vi "Reset (uSMC).vi"(7 "Timeout (sec)":dbl=10.0, 8 "error in":errorcluster, 9 "Index":i32, 10 "Reset Direction (false - towards maximal value)":bool, 11 "Visa Array In":refnum<visa-resource-name>[](array[refnum])) -> (0 "error out":errorcluster, 3 "Visa Array Out":refnum<visa-resource-name>[](array[refnum]))   [LabVIEW 2010, in "SignalWriterMH110203USBStepperMotor.lvclass"]
uses:
  SignalWriterMH110203USBStepperMotor.lvclass
  class_data.vi
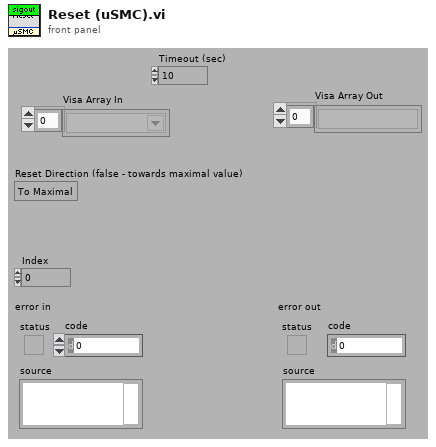
[diagram p1: front panel]
types:
  T1 = typedef "SignalWriterMH110203USBStepperMotor.lvclass/GoTo Control (uSMC).ctl" = cluster{"Step motor ID":string, "SMname":string, "Backlash":u16, "wait for input sygnal to start":bool, "use slow start/stop":bool, "units name":string, "Maximum speed":dbl, "speed":dbl, "step":u8, "point 1 ticks":i32, "point 2 ticks":i32, "point 1 units":dbl, "point 2 units":dbl, "Limit Switch standoff":dbl, "Zero Value":dbl, "Destination Position":dbl, "force backlash":bool, "power off when stop":bool, "POff delay":dbl, "positioner name":string, "R, Ohm":dbl, "I, mA":dbl, "Positioner's Type":u16, "Reset Direction":bool, "Manufacturer":string, "Model":string, "Scheme":string, "FirmwareVer":string}
  T2 = typedef "SignalWriterMH110203USBStepperMotor.lvclass/Get State Control (uSMC).ctl" = cluster{"Current Posistion":dbl, "CW/CCW":bool, "Speed":u16, "Temperature":dbl, "Power":u16, "Limit Switch 1":bool, "Limit Switch 2":bool, "After Reset":bool, "Step":u8, "Backlash":bool, "RT Error":bool, "RT State":bool, "Sync In":bool, "Sync Out":bool, "Ext Disconnect":bool, "Usb Powered":bool, "Voltage":dbl, "Working":bool, "SM Position in Encoder Units":i32, "Encoder Current Position":i32}
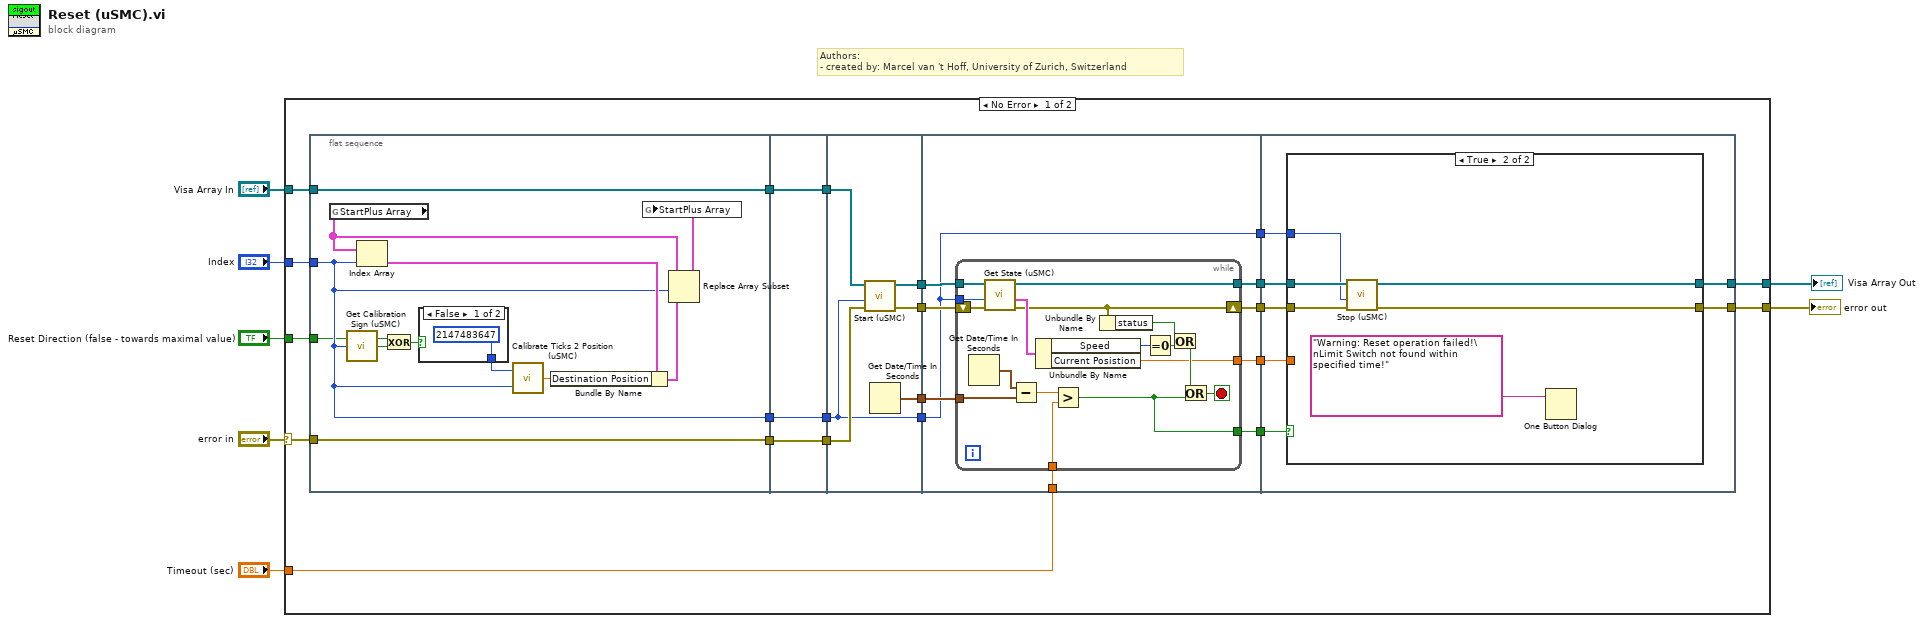
[diagram p0: block diagram]
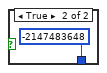
[diagram p2: hidden frame]
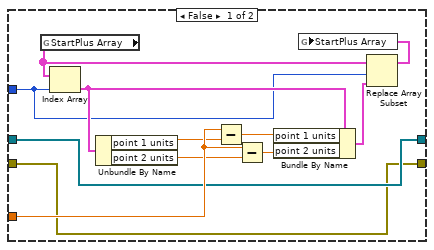
[diagram p3: hidden frame]
diagram:
  # "Authors: \n- created by: Marcel van 't Hoff, University of Zurich, Switzerland"
  n1 = case shown="No Error" "error in" {
    selector: "error in" -> [w8 w105]
    tunnel: "Index" -> [w14 _]
    tunnel: "Visa Array In" -> [w13 w104]
    tunnel: "Timeout (sec)" -> [w12 _]
    tunnel: "Reset Direction (false - towards maximal value)" -> [w11 _]
    tunnel: [w10 w104] -> w3
    tunnel: [w9 w105] -> w2
    frame No Error {
      n2 = flat-sequence {
        tunnel: w14 -> [w32]
        tunnel: w13 -> [w33]
        tunnel: [w33] -> w29
        tunnel: [w32] -> w28
        tunnel: [w31] -> w27
        tunnel: w8 -> [w31]
        tunnel: w11 -> [w30]
        tunnel: w29 -> [w46]
        tunnel: [w46] -> w26
        tunnel: w28 -> [w45]
        tunnel: [w45] -> w25
        tunnel: w27 -> [w44]
        tunnel: [w44] -> w24
        tunnel: w26 -> [w52]
        tunnel: w25 -> [w48]
        tunnel: w24 -> [w51]
        tunnel: [w50] -> w23
        tunnel: [w49] -> w22
        tunnel: [w48] -> w21
        tunnel: [w47] -> w20
        tunnel: w23 -> [w61]
        tunnel: w22 -> [w60]
        tunnel: w21 -> [w54]
        tunnel: w20 -> [w59]
        tunnel: w12 -> [w58]
        tunnel: [w57] -> w19
        tunnel: [w56] -> w18
        tunnel: [w55] -> w17
        tunnel: [w54] -> w16
        tunnel: [w53] -> w15
        tunnel: w19 -> [w85]
        tunnel: w18 -> [w81]
        tunnel: w17 -> [w82]
        tunnel: w16 -> [w84]
        tunnel: [w80] -> w10
        tunnel: w15 -> [w83]
        tunnel: [w79] -> w9
        frame #0 {
          n3 = global read "class_data.vi" "StartPlus Array"() -> (w35:T1[])
          n4 = call "Get Calibration Sign (uSMC).vi"("SM index"=w32) -> ("Calibration Sign"=w40:bool)  [unwired: 4 in]
          n5 = Index Array(array=w35, index=w32) -> (element=w41:T1)
          n6 = Exclusive Or(1:w40, 2:w30) -> (0:w39:bool)
          n7 = case shown="False" w39 {
            tunnel: [2147483647 ("ticks") -2147483648 ("ticks")] -> w38
            frame False {
            }
            frame True {
            }
          }
          n8 = call "Calibrate Ticks 2 Position (uSMC).vi"("array index"=w32, "ticks"=w38) -> ("value"=w37:dbl)
          n9 = Bundle By Name(cluster=w41, "Destination Position"=w37) -> (w36:T1)
          n10 = Replace Array Subset(array=w35, new element=w36, index=w32) -> (w34:T1[])
          n11 = global write "class_data.vi" "StartPlus Array"(w34) -> ()
        }
        frame #1 {
        }
        frame #2 {
          n12 = call "Start (uSMC).vi"("error in"=w51, "Index"=w48, "Visa Array In"=w52) -> ("error out"=w49:errorcluster, "Visa Array Out"=w50:refnum<visa-resource-name>[])  [unwired: 7 in]
          n13 = Get Date/Time In Seconds() -> (seconds since 1Jan1904=w47:timestamp)
        }
        frame #3 {
          n14 = while {
            tunnel: w61 -> [w78]
            tunnel: w54 -> [w76]
            tunnel: w59 -> [w72]
            tunnel: w58 -> [w70]
            shift-right: [w67] -> w56
            shift-left: w60 -> [w77]
            tunnel: [w68] -> w55
            tunnel: [w63] -> w57
            tunnel: [w62] -> w53
            stop <- w69 stop-if-true
            n15 = Get Date/Time In Seconds() -> (seconds since 1Jan1904=w73:timestamp)
            n16 = call "Get State (uSMC).vi"("error in (no error)"=w77, "SM number"=w76, "Visa array in"=w78) -> ("error out"=w67:errorcluster, "State cluster"=w75:T2, "Visa array out"=w68:refnum<visa-resource-name>[])  [unwired: 6 in]
            n17 = Subtract(x=w73, y=w72) -> (x-y=w71:dbl)
            n18 = Unbundle By Name(w75) -> ("Speed"=w74:u16, "Current Posistion"=w63:dbl)
            n19 = Greater?(x=w71, y=w70) -> (0:w62:bool)
            n20 = Unbundle By Name(w67) -> ("status"=w65:bool)
            n21 = Equal To 0?(x=w74) -> (x = 0?=w66:bool)
            n22 = Or(x=w65, y=w66) -> (x .or. y?=w64:bool)
            n23 = Or(x=w64, y=w62) -> (x .or. y?=w69:bool)
          }
        }
        frame #4 {
          n24 = case shown="True" w83 {
            tunnel: w85 -> [w97 _]
            tunnel: w84 -> [w91 w100]
            tunnel: w82 -> [w87 w102]
            tunnel: w81 -> [w86 w101]
            tunnel: [w87 w99] -> w80
            tunnel: [w86 w98] -> w79
            frame False {
              n25 = global read "class_data.vi" "StartPlus Array"() -> (w96:T1[])
              n26 = Index Array(array=w96, index=w91) -> (element=w95:T1)
              n27 = Unbundle By Name(w95) -> ("point 1 units"=w94:dbl, "point 2 units"=w93:dbl)
              n28 = Subtract(x=w97, y=w94) -> (x-y=w89:dbl)
              n29 = Subtract(x=w97, y=w93) -> (x-y=w88:dbl)
              n30 = Bundle By Name(cluster=w95, "point 1 units"=w89, "point 2 units"=w88) -> (w92:T1)
              n31 = Replace Array Subset(array=w96, new element=w92, index=w91) -> (w90:T1[])
              n32 = global write "class_data.vi" "StartPlus Array"(w90) -> ()
            }
            frame True {
              n33 = call "Stop (uSMC).vi"("error in (no error)"=w101, "Index"=w100, "Visa array in"=w102) -> ("error out"=w98:errorcluster, "Visa array out"=w99:refnum<visa-resource-name>[])  [unwired: 7 in]
              n34 = One Button Dialog(message="Warning: Reset operation failed!\nLimit Switch not found within specified time!") -> ()  [unwired: 1 in, 1 out]
            }
          }
        }
      }
    }
    frame Error {
    }
  }
  "error out" <- w2
  "Visa Array Out" <- w3
